vi "Node - Remove Channels.vi"(8 "error in (no error)":errorcluster, 10 "Node Ptr In":T1=18446744073709551615 format="%.0x", 11 "Compiled.Settings In":T2) -> (0 "error out":errorcluster, 2 "Node Ptr Out":T1=18446744073709551615 format="%.0x", 3 "Compiled.Settings Out":T2)   [LabVIEW 2016, in "PXImc Custom Device System Explorer.lvlib"]
uses:
  PXImc Custom Device System Explorer.lvlib
  Shared/Compiled.Settings.ctl
  <vilib>/NI Veristand/VeriStand Data/Byte Buffer/Byte Buffer.lvclass
  PXImc Router/Controls/Target Type.ctl
  PXImc Router/Controls/Router - Configuration.ctl
  PXImc Router/Controls/Router/Node Block R-W Properties.ctl
  PXImc Router/Controls/Router/Block Properties.ctl
  PXImc Router/Controls/Router/Router - PXImc Properties.ctl
  PXImc Router/Controls/Router/Router - PXImc Card Properties.ctl
  PXImc Router/Controls/Node Data.ctl
  PXImc Router/Controls/Node/Node - PXImc Parameters.ctl
  PXImc Router/Controls/Node/Node - Writer Data.ctl
  PXImc Router/Controls/Node/Node Ch Properties.ctl
  PXImc Router/Controls/Data Type.ctl
  PXImc Router/Controls/Node/Node - Readers Data.ctl
  PXImc Router/Controls/Node/Node - Reader Data.ctl
  <vilib>/NI Veristand/Custom Device API/Custom Device Item Ref.ctl
  Shared/Constants.vi
  <vilib>/NI VeriStand/Custom Device API/Custom Device API.lvlib
  Shared/PXImc Custom Device Shared.lvlib
  <vilib>/NI VeriStand/Custom Device Tools/Custom Device Utility Library/Custom Device Utility Library.lvlib
  PXImc Router/PXImc Router.lvlib
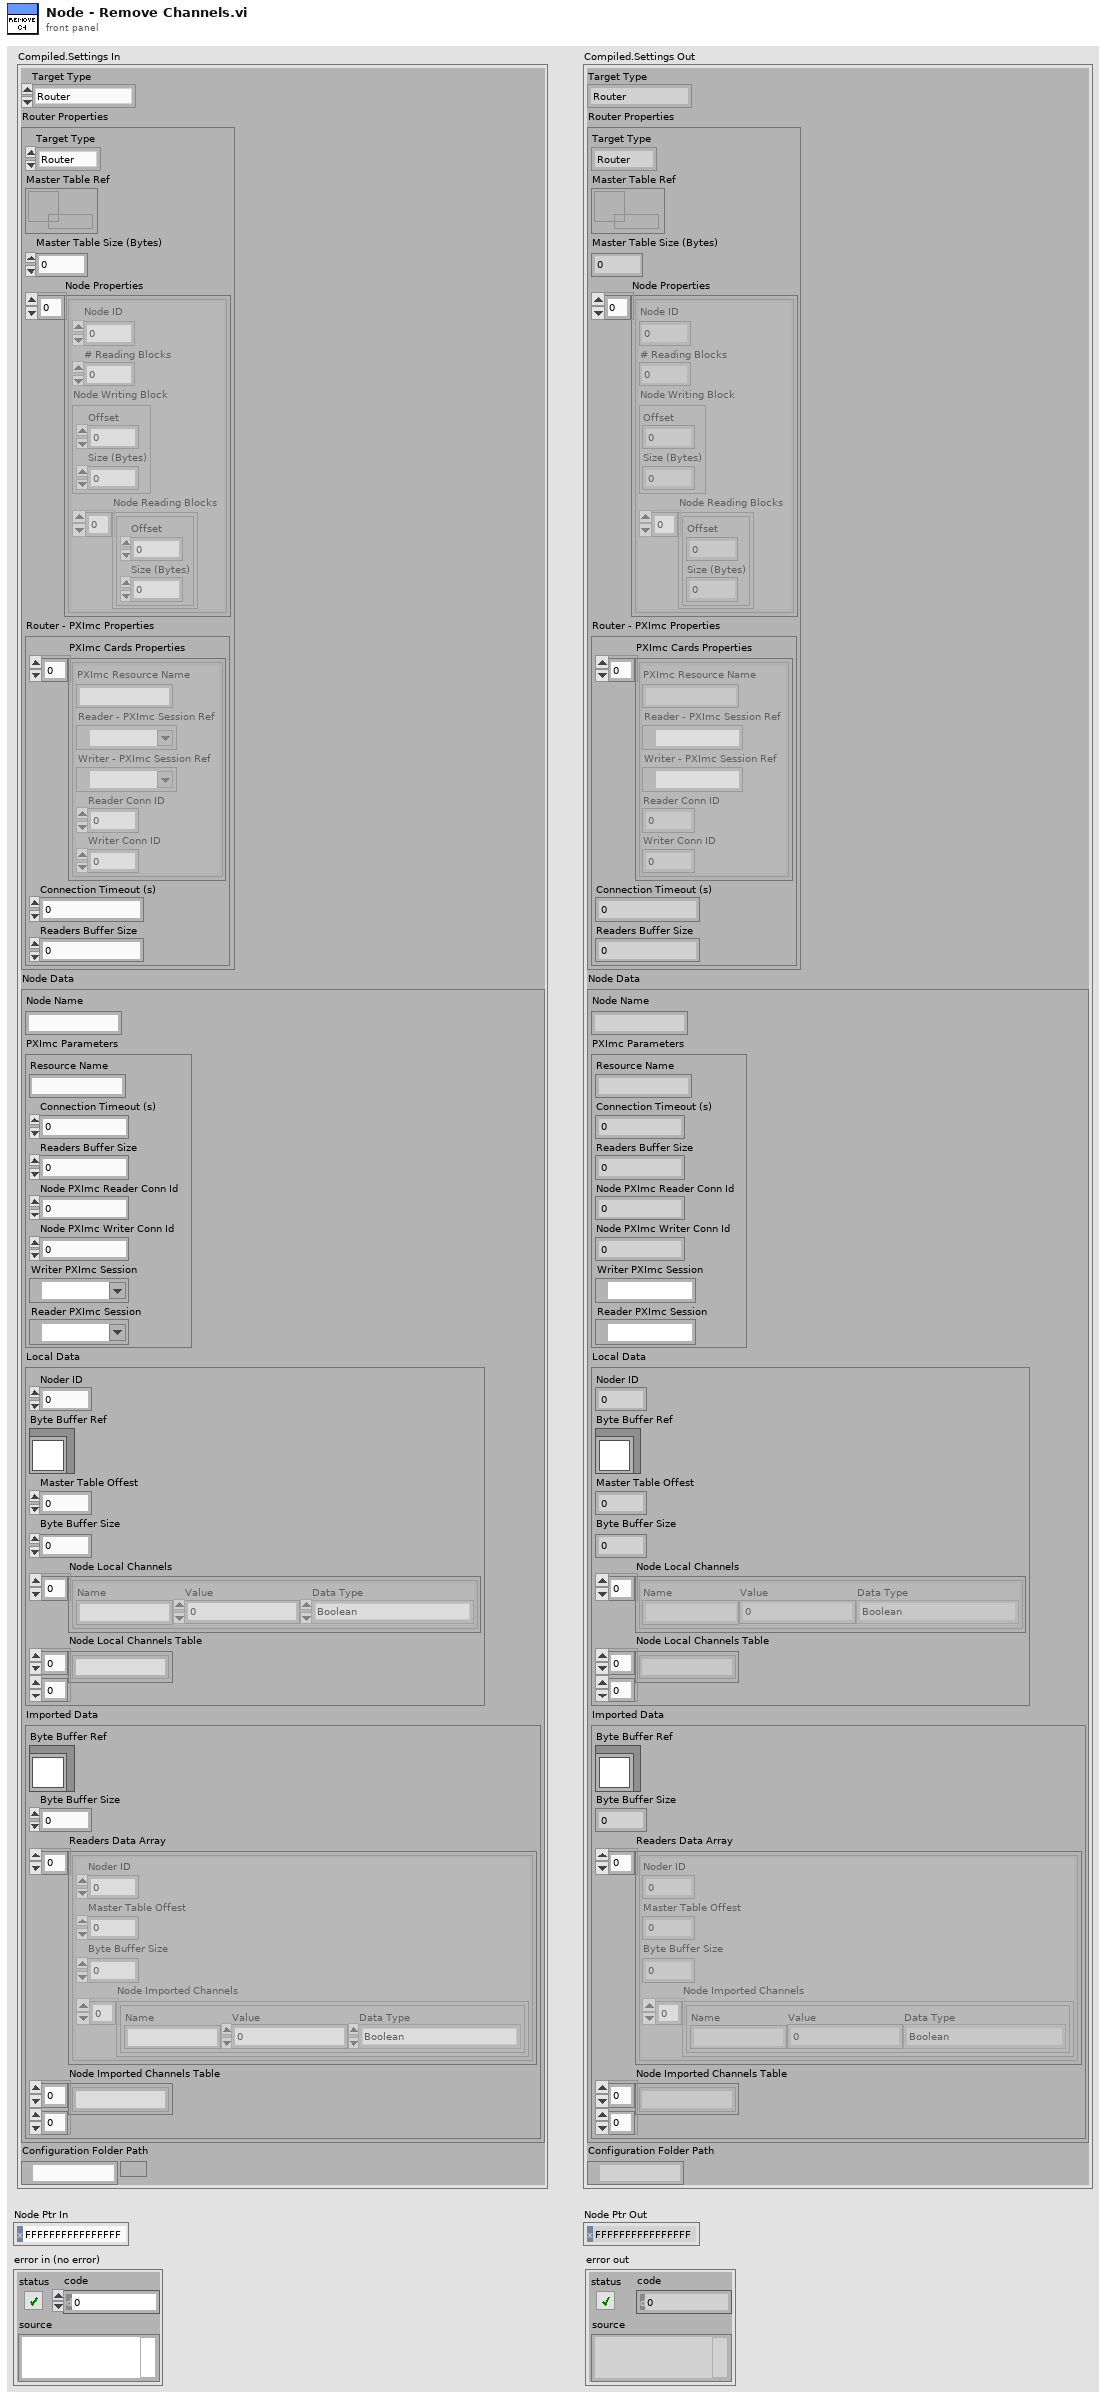
[diagram p1: front panel]
types:
  T1 = typedef "Custom Device API.lvlib/Custom Device Item Ref.ctl" = u64
  T2 = typedef "PXImc Custom Device Shared.lvlib/Compiled.Settings.ctl" = cluster{"Target Type":T3, "Router Properties":T4, "Node Data":T9, "Configuration Folder Path":path}
  T3 = typedef "PXImc Router.lvlib/Target Type.ctl" = enum16{"Router", "Node"}
  T4 = typedef "PXImc Router.lvlib/Router - Configuration.ctl" = cluster{"Target Type":T3, "Master Table Ref":refnum<data-value>, "Master Table Size (Bytes)":u32, "Node Properties":T5[], "Router - PXImc Properties":T7}
  T5 = typedef "PXImc Router.lvlib/Node Block R-W Properties.ctl" = cluster{"Node ID":u32, "# Reading Blocks":u32, "Node Writing Block":T6, "Node Reading Blocks":T6[]}
  T6 = typedef "PXImc Router.lvlib/Block Properties.ctl" = cluster{"Offset":u32, "Size (Bytes)":u32}
  T7 = typedef "PXImc Router.lvlib/Router - PXImc Properties.ctl" = cluster{"PXImc Cards Properties":T8[], "Connection Timeout (s)":dbl, "Readers Buffer Size":u64}
  T8 = typedef "PXImc Router.lvlib/Router - PXImc Card Properties.ctl" = cluster{"PXImc Resource Name":string, "Reader - PXImc Session Ref":refnum<k21>, "Writer - PXImc Session Ref":refnum<k21>, "Reader Conn ID":u16, "Writer Conn ID":u16}
  T9 = typedef "PXImc Router.lvlib/Node Data.ctl" = cluster{"Node Name":string, "PXImc Parameters":T10, "Local Data":T11, "Imported Data":T14}
  T10 = typedef "PXImc Router.lvlib/Node - PXImc Parameters.ctl" = cluster{"Resource Name":string, "Connection Timeout (s)":dbl, "Readers Buffer Size":u64, "Node PXImc Reader Conn Id":u16, "Node PXImc Writer Conn Id":u16, "Writer PXImc Session":refnum<k21>, "Reader PXImc Session":refnum<k21>}
  T11 = typedef "PXImc Router.lvlib/Node - Writer Data.ctl" = cluster{"Noder ID":u32, "Byte Buffer Ref":refnum<class "Byte Buffer.lvclass">, "Master Table Offest":u32, "Byte Buffer Size":u32, "Node Local Channels":T12[], "Node Local Channels Table":string[][]}
  T12 = typedef "PXImc Router.lvlib/Node Ch Properties.ctl" = cluster{"Name":string, "Value":dbl, "Data Type":T13}
  T13 = typedef "PXImc Router.lvlib/Data Type.ctl" = enum16{"Boolean", "SGL", "DBL", "I8", "I16", "I32", "I64", "U8", "U16", "U32", "U64"}
  T14 = typedef "PXImc Router.lvlib/Node - Readers Data.ctl" = cluster{"Byte Buffer Ref":refnum<class "Byte Buffer.lvclass">, "Byte Buffer Size":u64, "Readers Data Array":T15[], "Node Imported Channels Table":string[][]}
  T15 = typedef "PXImc Router.lvlib/Node - Reader Data.ctl" = cluster{"Noder ID":u32, "Master Table Offest":u32, "Byte Buffer Size":u64, "Node Imported Channels":T12[]}
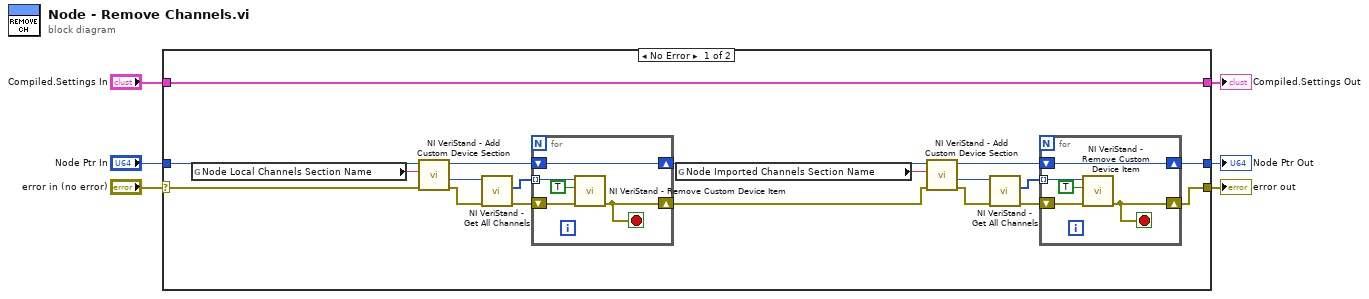
[diagram p0: block diagram]
diagram:
  n1 = case shown="No Error" "error in (no error)" {
    selector: "error in (no error)" -> [w23 w38]
    tunnel: [w10 w38] -> w3
    tunnel: "Node Ptr In" -> [w24 w37]
    tunnel: "Compiled.Settings In" -> [w25 w36]
    tunnel: [w9 w37] -> w1
    tunnel: [w25 w36] -> w4
    frame No Error {
      n2 = global read "Constants.vi" "Node Local Channels Section Name"() -> (w22:string)
      n3 = call <vilib>:"NI VeriStand - Add Custom Device Section.vi"("error in (no error)"=w23, "Section Name"=w22, "Parent Ref in"=w24) -> ("error out"=w20:errorcluster, "Section Ptr"=w21:T1, "Parent Ref out"=w18:T1)  [unwired: 5 in, 1 out]
      n4 = call <vilib>:"NI VeriStand - Get All Channels.vi"("error in"=w20, "Section Ref in"=w21) -> ("error out"=w19:errorcluster, "Channel Refs"=w8:T1[])  [unwired: 6 in, 2 out]
      n5 = for {
        shift-right: [w28] -> w12
        shift-left: w18 -> [w28]
        shift-right: [w27] -> w11
        shift-left: w19 -> [w29]
        tunnel: w8 -> [w26] mode=indexing
        stop <- w27 stop-if-true
        n6 = call <vilib>:"NI VeriStand - Remove Custom Device Item.vi"("error in (no error)"=w29, "Force Delete (F)"=TRUE, "Item Ref in"=w26) -> ("error out"=w27:errorcluster)  [unwired: 7 in, 1 out]
      }
      n7 = global read "Constants.vi" "Node Imported Channels Section Name"() -> (w13:string)
      n8 = call <vilib>:"NI VeriStand - Add Custom Device Section.vi"("error in (no error)"=w11, "Section Name"=w13, "Parent Ref in"=w12) -> ("error out"=w15:errorcluster, "Section Ptr"=w14:T1, "Parent Ref out"=w17:T1)  [unwired: 5 in, 1 out]
      n9 = call <vilib>:"NI VeriStand - Get All Channels.vi"("error in"=w15, "Section Ref in"=w14) -> ("error out"=w16:errorcluster, "Channel Refs"=w7:T1[])  [unwired: 6 in, 2 out]
      n10 = for {
        tunnel: w7 -> [w34] mode=indexing
        shift-right: [w32] -> w9
        shift-left: w17 -> [w32]
        shift-right: [w31] -> w10
        shift-left: w16 -> [w33]
        stop <- w31 stop-if-true
        n11 = call <vilib>:"NI VeriStand - Remove Custom Device Item.vi"("error in (no error)"=w33, "Force Delete (F)"=TRUE, "Item Ref in"=w34) -> ("error out"=w31:errorcluster)  [unwired: 7 in, 1 out]
      }
    }
    frame Error {
    }
  }
  "Compiled.Settings Out" <- w4
  "error out" <- w3
  "Node Ptr Out" <- w1
